vi "Scale triangle.vi"(1 "Scale factors (Sx, Sy, Sz)":sgl[](array[numeric]), 2 "Triangle in":T1) -> (0 "Triangle out":T1)   [LabVIEW 2014]
uses:
  Typedefs/Triangle.ctl
  <vilib>/Analysis/baseanly.llb/A x Vector.vi
  <vilib>/Analysis/NI_AALBase.lvlib
panel:
  # "PN 13/01/2015"
  # "Vertices"
  # "Edges"
  # "Unit normal"
  # "pre-store"
  # "Vertices"
  # "Edges"
  # "Unit normal"
  # "pre-store"
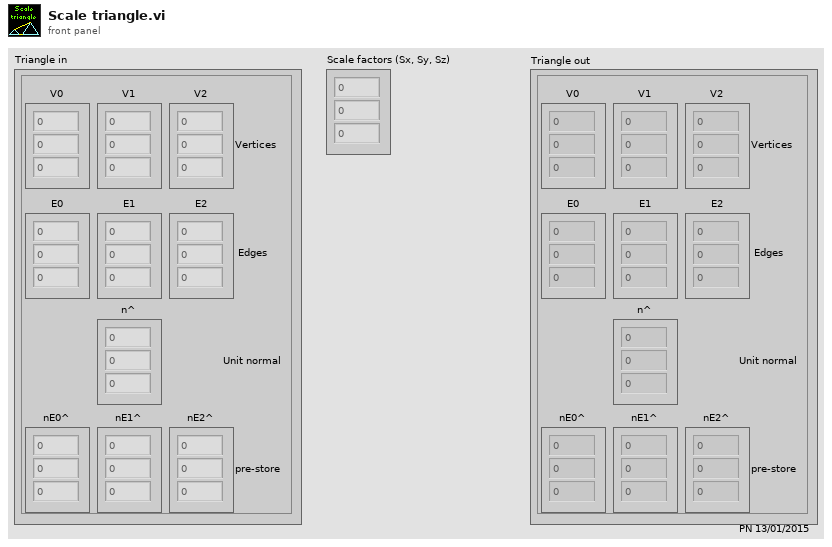
[diagram p1: front panel]
types:
  T1 = typedef "Triangle.ctl" = cluster{"V0":sgl[], "V1":sgl[], "V2":sgl[], "E0":sgl[], "E1":sgl[], "E2":sgl[], "n^":sgl[], "nE0^":sgl[], "nE1^":sgl[], "nE2^":sgl[]}
  T2 = typedef "NI_Matrix.lvlib/RealMatrix.ctl" = dbl[][]
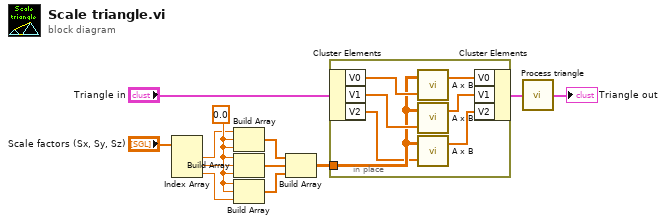
[diagram p0: block diagram]
diagram:
  w10 = sgl 0.0
  n1 = Index Array(array="Scale factors (Sx, Sy, Sz)") -> (element #1=w9:sgl, element #2=w8:sgl, element #3=w7:sgl)  [unwired: 3 in]
  n2 = Build Array(w9, w10, w10) -> (w6:sgl[])
  n3 = Build Array(w10, w8, w10) -> (w5:sgl[])
  n4 = Build Array(w10, w10, w7) -> (w4:sgl[])
  n5 = Build Array(w6, w5, w4) -> (w3:T2)
  n6 = in-place {
    in-place-border: w3 -> [w16]
    n7 = in-place-cluster #1("Triangle in") -> ("V0"=w19:sgl[], "V1"=w17:sgl[], "V2"=w15:sgl[])
    n8 = call-poly <vilib>:"A x B.vi"("Vector"=w19, "A"=w16) -> ("A x Vector"=w18:dbl[])  [unwired: 1 out]
    n9 = call-poly <vilib>:"A x B.vi"("Vector"=w17, "A"=w16) -> ("A x Vector"=w14:dbl[])  [unwired: 1 out]
    n10 = call-poly <vilib>:"A x B.vi"("Vector"=w15, "A"=w16) -> ("A x Vector"=w13:dbl[])  [unwired: 1 out]
    n11 = in-place-cluster #1("V0"=w18, "V1"=w14, "V2"=w13) -> (w2:T1)
  }
  n12 = call "Process triangle.vi"("Triangle in"=w2) -> ("Triangle out"=→"Triangle out":T1)
